vi "ROI entry-Get line mode value.vi"(8 "error in (no error)":errorcluster) -> (0 "error out":errorcluster, 3 "Drawing Mode setting":T1=enum."Orthogonal")   [LabVIEW 2013]
uses:
  Typedefs/Line draw mode.ctl
  ROI Entry screen/Globals/gl_ROI Entry UI globals.vi
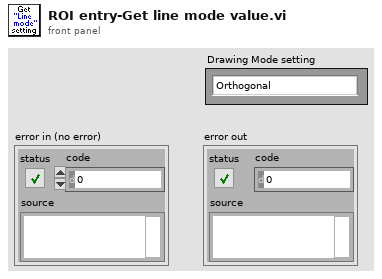
[diagram p1: front panel]
types:
  T1 = typedef "Line draw mode.ctl" = enum16{"Free draw", "Orthogonal"}
  T2 = typedef "ROI entry screen ctrl refs cluster.ctl" = cluster{"Done button":refnum<vi>, "Imaging button":refnum<vi>, "Acquisition button":refnum<vi>, "POI dwell time (us)":refnum<vi>, "Scan dwell time per pixel (us)":refnum<vi>, "# of planes":refnum<vi>, "Zoom":refnum<vi>, "Equal size":refnum<vi>, "Channel":refnum<vi>, "Image Display":refnum<vi>, "Z-Plane Selector":refnum<vi>, "Number of lines left":refnum<vi>, "Z-stack folder path":refnum<vi>, "POI Density":refnum<vi>, "Arb Plane Entry":refnum<vi>, "Whole plane":refnum<vi>, "Clear Last":refnum<vi>, "Clear All":refnum<vi>, "Trial Length (sec)":refnum<vi>, "Palette Type":refnum<vi>, "Intensity slider":refnum<vi>, "# POI":refnum<vi>, "Max Z Proj":refnum<vi>, "Zplane ind":refnum<vi>, "Wavelength (nm)":refnum<vi>, "Number of Trials":refnum<vi>, "Funct stim.trig.enable":refnum<vi>, "Funct stim.trig.delay (s)":refnum<vi>, "Line Mode":refnum<vi>, "Step size (µm)":refnum<vi>, "ROI move mode":refnum<vi>, "Cool-down time (s)":refnum<vi>, "Enable cool-down time":refnum<vi>, "Motor Z ind. (um)":refnum<vi>, "AOL Z ind. (um)":refnum<vi>}
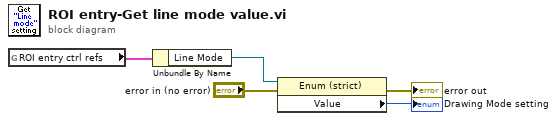
[diagram p0: block diagram]
diagram:
  n1 = global read "gl_ROI Entry UI globals.vi" "ROI entry ctrl refs"() -> (w5:T2)
  n2 = Unbundle By Name(w5) -> ("Line Mode"=w4:refnum<vi>)
  n3 = property on="Property Node" class="Enum (strict)"(reference=w4, error in="error in (no error)") -> (error out=→"error out":errorcluster, "Value"=→"Drawing Mode setting":T1)  [unwired: 1 out]
